vi "Configure Limit Testing.vi"(0 "VISA resource name":refnum<visa-resource-name>, 1 "limit test (T)":bool=TRUE, 2 "lower limit (T)":bool=TRUE, 3 "lower limit (0)":dbl min=-9.9e+37 max=9.9e+37 step=1.0 format="%.3e", 5 "limit test function (1:One)":u16(ring)=1 items=["One"=1, "Two"=2], 7 "comparator beeper (T)":bool=TRUE, 9 "beeper mode (0:fail)":u16(ring) items=["Beep on fail", "Beep on pass"], 11 "error in (no error)":errorcluster, 12 "upper limit (T)":bool=TRUE, 13 "upper limit (1.000E+5)":dbl=100000.0 min=-9.9e+37 max=9.9e+37 step=1.0 format="%.3e") -> (4 "VISA resource name out":refnum<visa-resource-name>, 15 "error out":errorcluster)   [LabVIEW 2016, in "Agilent 4263X.lvlib"]
doc: "This VI configures the limit testing features of the instrument."
uses:
  <instrlib>/Agilent 4263X/Agilent 4263X.lvlib
panel:
  # "limit test parameters"
  # "on ------------>\noff"
  # "on ------------->\noff"
  # "on ------------>\noff"
  # "on ------------>\noff"
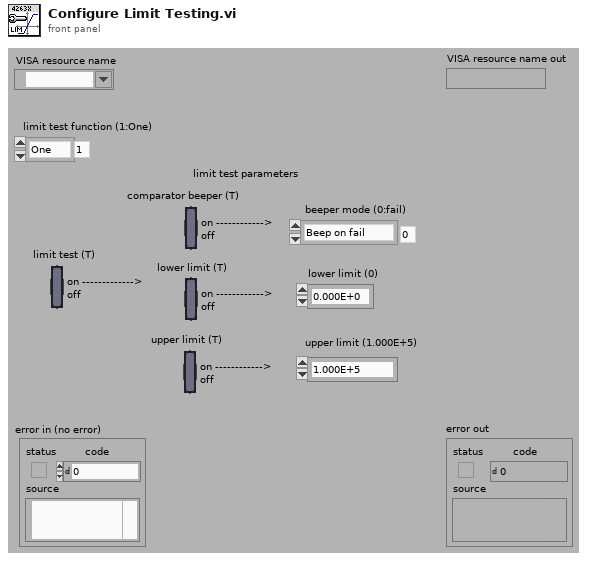
[diagram p1: front panel]
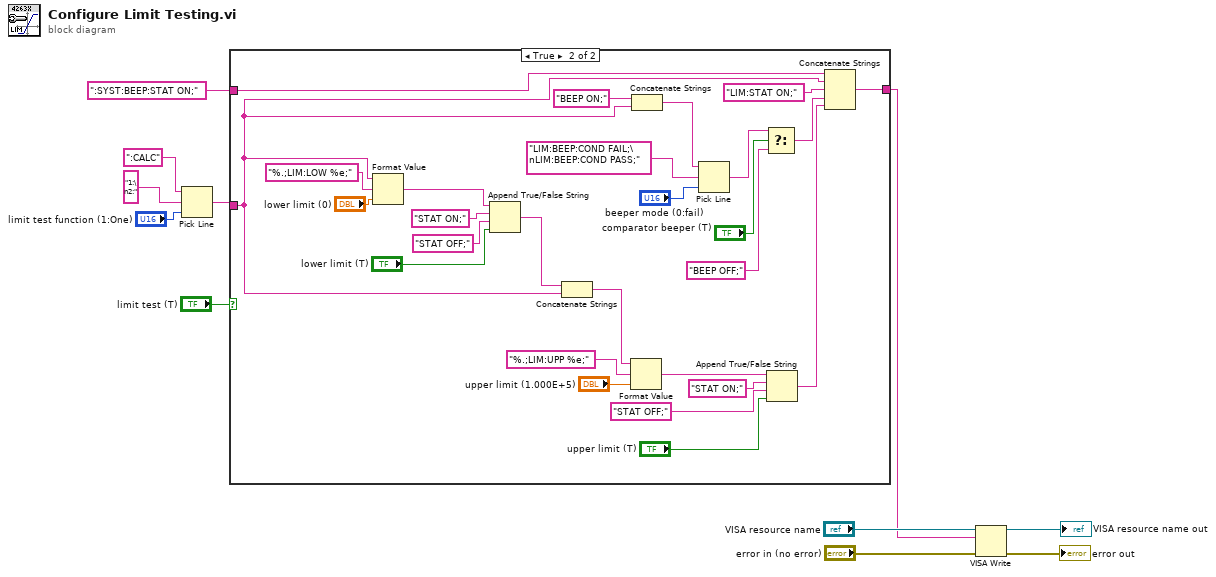
[diagram p0: block diagram]
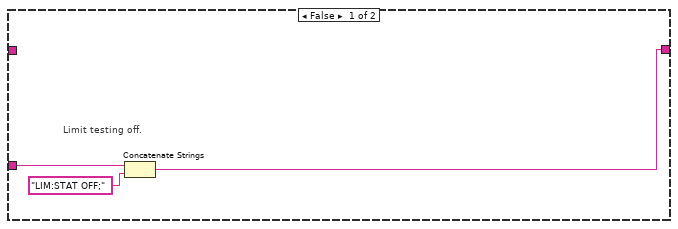
[diagram p2: hidden frame]
diagram:
  n1 = Pick Line(string ("")=":CALC", multi-line string="1:\n2:", line index="limit test function (1:One)") -> (output string=w6:string)
  n2 = case shown="True" "limit test (T)" {
    tunnel: w6 -> [w14 w21]
    tunnel: [w12 w23] -> w5
    tunnel: ":SYST:BEEP:STAT ON;" -> [_ w17]
    frame False {
      # "Limit testing off."
      n3 = Concatenate Strings(w14, "LIM:STAT OFF;") -> (w12:string)
    }
    frame True {
      n4 = Format Value(string ("")=w21, format string="%.;LIM:LOW %e;", value (0)="lower limit (0)") -> (output string=w32:string)
      n5 = Append True/False String(1:"lower limit (T)", 2:"STAT OFF;", 3:"STAT ON;", 4:w32) -> (0:w20:string)
      n6 = Concatenate Strings(w20, w21) -> (w19:string)
      n7 = Format Value(string ("")=w19, format string="%.;LIM:UPP %e;", value (0)="upper limit (1.000E+5)") -> (output string=w26:string)
      n8 = Concatenate Strings("BEEP ON;", w21) -> (w15:string)
      n9 = Pick Line(string ("")=w15, multi-line string="LIM:BEEP:COND FAIL;\nLIM:BEEP:COND PASS;", line index="beeper mode (0:fail)") -> (output string=w39:string)
      n10 = Select(t=w39, s="comparator beeper (T)", f="BEEP OFF;") -> (s? t:f=w24:string)
      n11 = Append True/False String(1:"upper limit (T)", 2:"STAT OFF;", 3:"STAT ON;", 4:w26) -> (0:w18:string)
      n12 = Concatenate Strings(w17, w21, "LIM:STAT ON;", w24, w18) -> (w23:string)
    }
  }
  n13 = VISA Write(VISA resource name="VISA resource name", write buffer=w5, error in (no error)="error in (no error)") -> (VISA resource name out=→"VISA resource name out":refnum<visa-resource-name>, error out=→"error out":errorcluster)  [unwired: 1 out]
